vi "F1240_SP_FileMerger.vi"() -> ()   [LabVIEW 2018]
uses:
  <vilib>/Utility/file.llb/Read From Spreadsheet File (string).vi
  <vilib>/Utility/file.llb/Write To Spreadsheet File (string).vi
panel:
  in  "Write to File(T)":bool=TRUE
  in  "Merged Filename":path
  in  "Source Folder":path=path "\\\\Tyn2ua1211mwr\\c/IdtATE/Results/F1241_SP_NSN_SAMPLES_0711/Processed IPE Data/Raw Data"
  out "Header":string
  out "all rows 2":string[][](array[string])
  out "all rows":string[][](array[string])
  out "Channel":string[](array[string])
  out "SN":string[](array[string])
  out "filenames":string[](array[string])
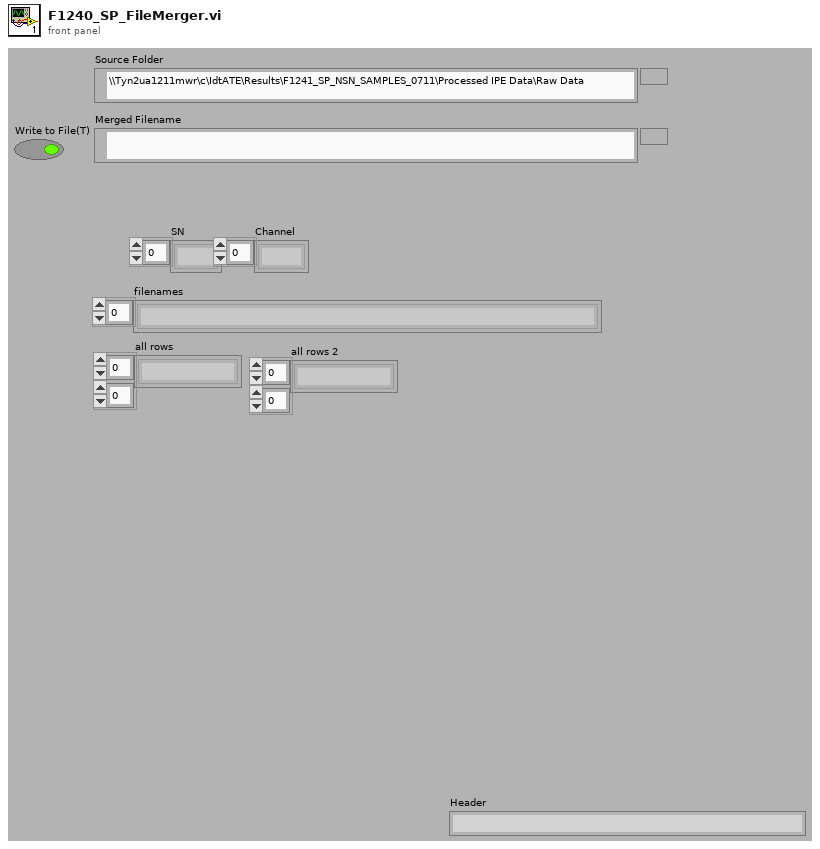
[diagram p1: front panel]
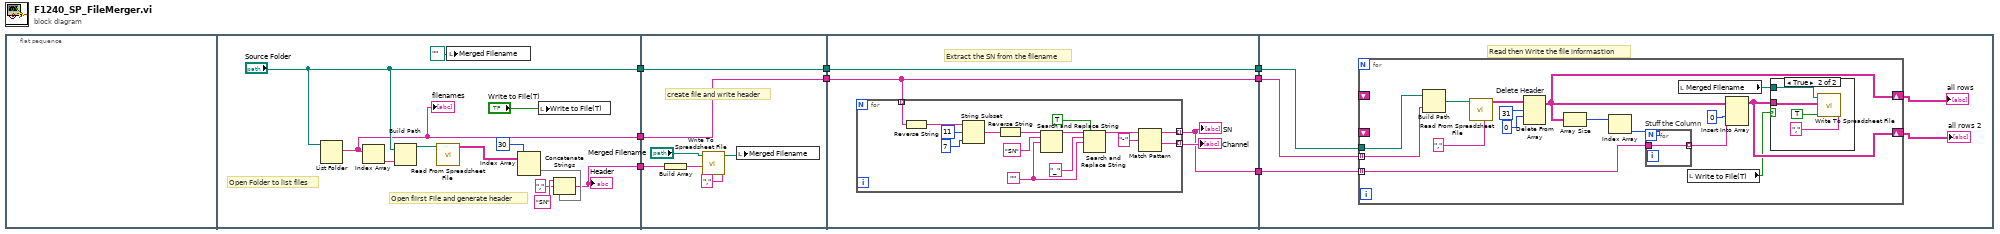
[diagram p0: block diagram]
diagram:
  n1 = flat-sequence {
    tunnel: [w11] -> w8
    tunnel: ["Source Folder"] -> w7
    tunnel: [w12] -> w6
    tunnel: w8 -> [w27]
    tunnel: w7 -> [w26]
    tunnel: w6 -> [w24]
    tunnel: [w27] -> w5
    tunnel: [w26] -> w4
    tunnel: w5 -> [w28]
    tunnel: w4 -> [w31]
    tunnel: [w28] -> w3
    tunnel: [w31] -> w2
    tunnel: [w29] -> w1
    tunnel: w3 -> [w50]
    tunnel: w2 -> [w49]
    tunnel: w1 -> [w51]
    frame #0 {
    }
    frame #1 {
      # "Open fiirst File and generate header"
      # "Open Folder to list files"
      n2 = List Folder(path="Source Folder") -> (filenames=w11:string[])  [unwired: 3 in, 3 out]
      "filenames" <- w11
      n3 = Index Array(array=w11) -> (element=w20:string)  [unwired: 1 in]
      n4 = Build Path(base path="Source Folder", name or relative path=w20) -> (appended path=w18:path)
      n5 = call-poly <vilib>:"Read From Spreadsheet File.vi"("file path (dialog if empty)"=w18) -> ("all rows"=w17:string[][])  [unwired: 6 in, 4 out]
      n6 = local write "Merged Filename"(path "" ("Merged Filename")) -> ()
      n7 = Index Array(array=w17, index (row)=30 ("index (row) 2")) -> (element=w13:string[])  [unwired: 1 in]
      n8 = local write "Write to File(T)"("Write to File(T)") -> ()
      n9 = Concatenate Strings("SN" ("new element/subarray"), "," ("string"), w13) -> (w12:string)
      "Header" <- w12
    }
    frame #2 {
      # "create file and write header"
      n10 = Build Array(w24) -> (w23:string[])
      n11 = call-poly <vilib>:"Write To Spreadsheet File.vi"("delimiter (\\t)"="," ("delimiter (\\t)"), "1D data"=w23, "file path (dialog if empty)"="Merged Filename") -> ("new file path (Not A Path if cancelled)"=w21:path)  [unwired: 5 in]
      n12 = local write "Merged Filename"(w21) -> ()
    }
    frame #3 {
      # "Extract the SN from the filename"
      n13 = for {
        tunnel: [w34] -> w29 mode=indexing
        tunnel: [w33] -> w30 mode=indexing
        tunnel: w28 -> [w32] mode=indexing
        w38 = ""
        n14 = Reverse String(1:w32) -> (0:w43:string)
        n15 = String Subset(string=w43, offset (0)=11, length (rest)=7 ("length (rest)")) -> (substring=w46:string)
        n16 = Reverse String(1:w46) -> (0:w42:string)
        n17 = Search and Replace String(input string=w42, search string="SN", replace string=w38) -> (result string=w40:string)  [unwired: 5 in, 3 out]
        n18 = Search and Replace String(replace all?=TRUE ("replace all? (F)"), input string=w40, search string="_", replace string=w38) -> (result string=w36:string)  [unwired: 4 in, 3 out]
        n19 = Match Pattern(string=w36, regular expression="-") -> (before substring=w34:string, after substring=w33:string)  [unwired: 1 in, 2 out]
      }
      "Channel" <- w30
      "SN" <- w29
    }
    frame #4 {
      # "Read then Write the file informastion"
      n20 = for {
        tunnel: w50 -> [w66] mode=indexing
        tunnel: w49 -> [w65]
        shift-right: [w57] -> w47
        shift-left: _ -> [_]
        tunnel: w51 -> [w59] mode=indexing
        shift-right: [w54] -> w48
        shift-left: _ -> [_]
        n21 = Build Path(base path=w65, name or relative path=w66) -> (appended path=w67:path)
        n22 = call-poly <vilib>:"Read From Spreadsheet File.vi"("delimiter (\\t)"="," ("delimiter (\\t)"), "file path (dialog if empty)"=w67) -> ("all rows"=w63:string[][])  [unwired: 5 in, 4 out]
        n23 = Delete From Array "Delete Header"(array=w63, length=31, index (row)=0) -> (array with subset deleted=w57:string[][])  [unwired: 1 in, 1 out]
        n24 = Array Size(array=w57) -> (size(s)=w60:i32[])
        n25 = Index Array(array=w60) -> (element=w58:i32)  [unwired: 1 in]
        n26 = for "Stuff the Column" {
          N: w58 -> [_]
          tunnel: w59 -> [w72]
          tunnel: [w72] -> w56 mode=indexing
        }
        n27 = local read "Merged Filename"() -> (w52:path)
        n28 = local read "Write to File(T)"() -> (w53:bool)
        n29 = Insert Into Array(array=w57, index (col)=0 ("disabled index (col)"), new element=w56) -> (w54:string[][])  [unwired: 1 in]
        n30 = case shown="True" w53 {
          tunnel: w54 -> [_ w71]
          tunnel: w52 -> [_ w68]
          frame False {
          }
          frame True {
            n31 = call-poly <vilib>:"Write To Spreadsheet File.vi"("delimiter (\\t)"="," ("delimiter (\\t)"), "append to file? (new file:F)"=TRUE, "2D data"=w71, "file path (dialog if empty)"=w68) -> ()  [unwired: 4 in, 1 out]
          }
        }
      }
      "all rows" <- w47
      "all rows 2" <- w48
    }
  }
